vi "_Event Notification.Test.vi"() -> ()   [LabVIEW 2024, in "EQMF.lvlib" / "Event Log.lvlib"]
uses:
  Event Log.lvlib
  Event Log.Log Level.ctl
  Event Log.Notification Type.ctl
  Event Notification.lvclass
  Queues/Queue Utils.lvlib
panel:
  in  "Clear Status":bool
  in  "Type":T1
  in  "Logging Level":T2
  in  "Msg Level":T2
  in  "Display":bool
  in  "Log":bool
  in  "stop":bool
  out "Status":string
  in  "error in":errorcluster
  in  "Reset Logged":bool
  out "Logged":bool
  in  "Event + Error":bool
  in  "Event":bool
  in  "Event Msg":string
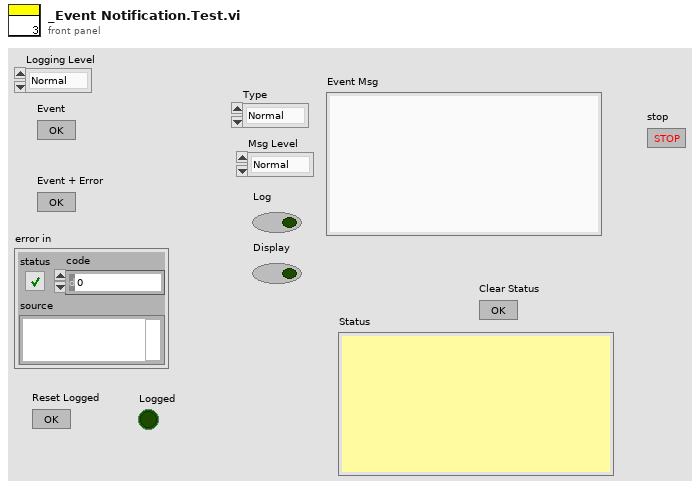
[diagram p1: front panel]
types:
  T1 = typedef "EQMF.lvlib/Event Log.lvlib/Event Log.Notification Type.ctl" = enum16{"Normal", "Warning", "Error", "Success"}
  T2 = typedef "EQMF.lvlib/Event Log.lvlib/Event Log.Log Level.ctl" = enum16{"Normal", "Verbose", "Debug0", "Debug1", "Debug2"}
  T3 = typedef "EQMF.lvlib/Queue Utils.lvlib/Q.Element.ctl" = cluster{"Cmd":string, "Sub":string, "Data1":variant, "Data2":variant}
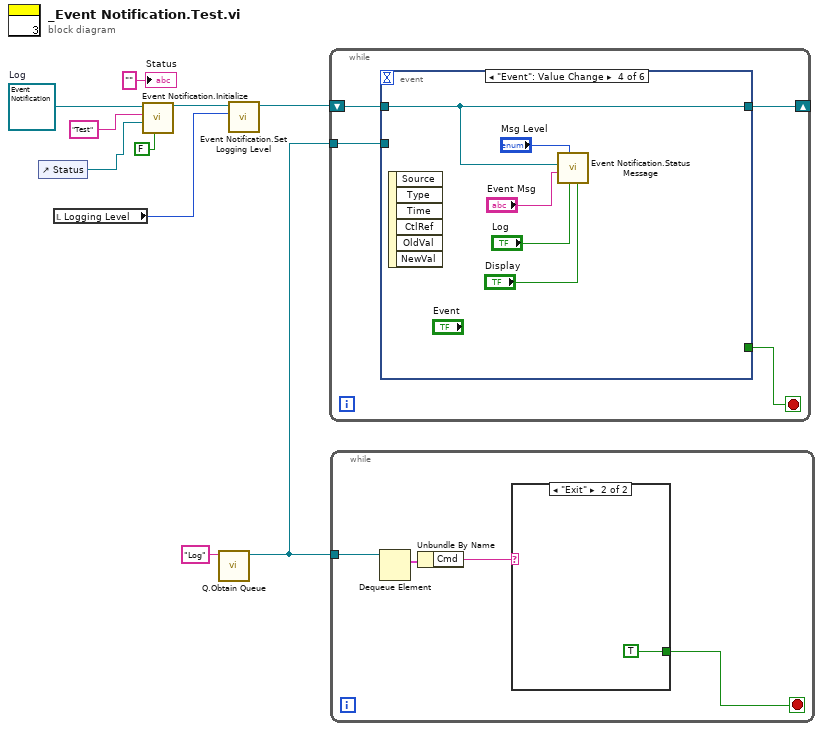
[diagram p0: block diagram]
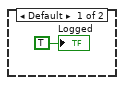
[diagram p2: hidden frame]
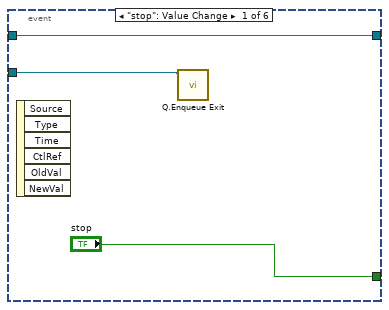
[diagram p3: hidden frame]
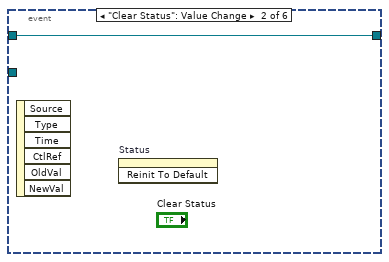
[diagram p4: hidden frame]
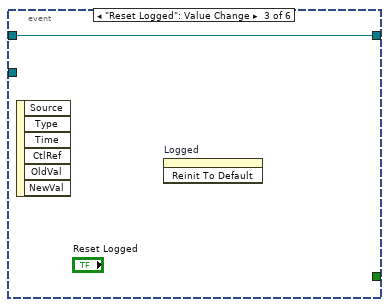
[diagram p5: hidden frame]
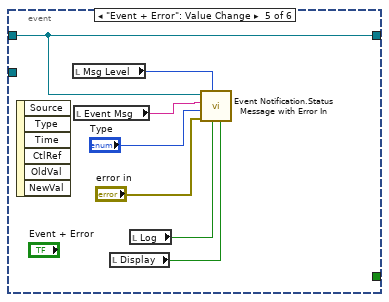
[diagram p6: hidden frame]
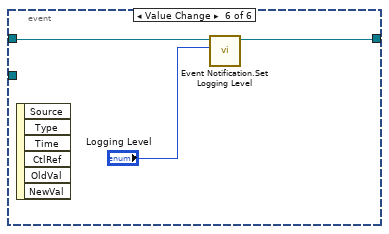
[diagram p7: hidden frame]
diagram:
  w8 = refnum<class "Event Notification.lvclass"> refnum  # Log
  n1 = control-ref of="Status"() -> (w5:refnum<vi>)
  n2 = local read "Logging Level"() -> (w1:T2)
  n3 = call "Event Notification.Initialize.vi"("Is Child?"=FALSE, "StatusTxtBoxRef"=w5, "AppID"="Test", "Event Notification in"=w8) -> ("Event Notification out"=w3:refnum<class "Event Notification.lvclass">)  [unwired: 6 in, 1 out]
  n4 = call "Q.Obtain Queue.vi"("Q Name"="Log") -> ("Q Out"=w9:refnum<queue>)  [unwired: 8 in, 2 out]
  n5 = call "Event Notification.Set Logging Level.vi"("Log Level"=w1, "Event Notification in"=w3) -> ("Event Notification out"=w2:refnum<class "Event Notification.lvclass">)  [unwired: 9 in]
  n6 = while {
    tunnel: w9 -> [w13]
    shift-right: [w11] -> _
    shift-left: w2 -> [w12]
    stop <- w14 stop-if-true
    n7 = event shown="[3] \"Event\": Value Change" {
      selector: _ -> [_ _ _ _ _ _]
      dyn-events: _ -> [_ _ _ _ _ _]
      timeout: _ -> [_ _ _ _ _ _]
      tunnel: ["stop" _ _ _ _ _] -> w14
      tunnel: w13 -> [w16 _ _ _ _ _]
      tunnel: w12 -> [w15 w18 w19 w24 w25 w34]
      tunnel: [w15 w18 w19 w24 w25 w32] -> w11
      event "stop": Value Change {
        n8 = event-data() -> ()  [unwired: 1 in, 6 out]
        n9 = call "Q.Enqueue Exit.vi"("Q In"=w16) -> ()  [unwired: 9 in, 2 out]
      }
      event "Clear Status": Value Change {
        n10 = event-data() -> ()  [unwired: 1 in, 6 out]
        n11 = invoke on="Status" class="Str" method="Reinit To Default"() -> ()  [unwired: 3 in, 3 out]
      }
      event "Reset Logged": Value Change {
        n12 = event-data() -> ()  [unwired: 1 in, 6 out]
        n13 = invoke on="Logged" class="Bool (strict)" method="Reinit To Default"() -> ()  [unwired: 3 in, 3 out]
      }
      event "Event": Value Change {
        n14 = event-data() -> ()  [unwired: 1 in, 6 out]
        n15 = call "Event Notification.Status Message.vi"("Display"="Display", "Log"="Log", "Level"="Msg Level", "Message"="Event Msg", "Event Notification in"=w24) -> ()  [unwired: 7 in]
      }
      event "Event + Error": Value Change {
        n16 = event-data() -> ()  [unwired: 1 in, 6 out]
        n17 = local read "Msg Level"() -> (w31:T2)
        n18 = local read "Event Msg"() -> (w30:string)
        n19 = local read "Display"() -> (w27:bool)
        n20 = local read "Log"() -> (w28:bool)
        n21 = call "Event Notification.Status Message with Error In.vi"("Display"=w27, "Log"=w28, "Level"=w31, "Error"="error in", "Type"="Type", "Message"=w30, "Event Notification in"=w25) -> ()  [unwired: 5 in]
      }
      event Value Change {
        n22 = event-data() -> ()  [unwired: 1 in, 6 out]
        n23 = call "Event Notification.Set Logging Level.vi"("Log Level"="Logging Level", "Event Notification in"=w34) -> ("Event Notification out"=w32:refnum<class "Event Notification.lvclass">)  [unwired: 9 in]
      }
    }
  }
  n24 = while {
    tunnel: w9 -> [w38]
    stop <- w35 stop-if-true
    n25 = Dequeue Element(queue=w38) -> (element=w37:T3)  [unwired: 2 in, 3 out]
    n26 = Unbundle By Name(w37) -> ("Cmd"=w36:string)
    n27 = case shown="\"Exit\"" w36 {
      tunnel: [_ TRUE] -> w35
      frame Default {
        "Logged" <- TRUE ("Logged")
      }
      frame "Exit" {
      }
    }
  }
  "Status" <- "" ("Status")
